vi "test_read-nmea-data2.vi"() -> ()   [LabVIEW 2019] (continued)
\n15:12:28.01\tF9P\t\t\n15:12:28.03\tF9P\t\t\n15:12:28.05\tF9P\t\t\n15:12:28.07\tF9P\t\t\n15:12:28.09\tF9P\t\t\n15:12:28.11\tF9P\t\t\n15:12:28.13\tF9P\t\t\n15:12:28.15\tF9P\t\t\n15:12:28.17\tF9P\t\t\n15:12:28.19\tF9P\t\t\n15:12:28.21\tF9P\t\t\n15:12:28.23\tF9P\t$GNRMC,061230.00,A,3723.54055,N,12656.94219,E,1.668,58.60,250720,,,A,V*39\n\t\n15:12:28.25\tF9P\t$GNVTG,58.60,T,,M,1.668,N,3.089,K,A*13\n\t\n15:12:28.27\tF9P\t$GNGGA,061230.00,3723.54055,N,12656.94219,E,1,12,0.92,43.1,M,18.5,M,,*73\n\t\n15:12:28.29\tF9P\t$GNGSA,A,3,12,06,19,05,17,09,04,02,,,,,1.52,0.92,1.22,1*0C\n\t\n15:12:28.31\tF9P\t$GNGSA,A,3,85,70,71,84,,,,,,,,,1.52,0.92,1.22,2*0E\n\t\n15:12:28.33\tF9P\t$GNGSA,A,3,36,19,11,04,09,12,,,,,,,1.52,0.92,1.22,3*0C\n\t\n15:12:28.35\tF9P\t$GNGSA,A,3,14,11,33,,,,,,,,,,1.52,0.92,1.22,4*0D\n\t\n15:12:28.37\tF9P\t$GPGSV,3,1,09,02,55,319,20,04,18,043,27,05,37,247,33,06,64,049,30,1*61\n\t\n15:12:28.39\tF9P\t$GPGSV,3,2,09,09,45,074,31,12,23,276,31,17,33,154,37,19,52,157,32,1*69\n\t\n15:12:28.41\tF9P\t$GPGSV,3,3,09,25,12,306,,1*5C\n\t\n15:12:28.43\tF9P\t$GPGSV,3,1,09,02,55,319,,04,18,043,21,05,37,247,26,06,64,049,26,6*61\n\t\n15:12:28.45\tF9P\t$GPGSV,3,2,09,09,45,074,25,12,23,276,17,17,33,154,31,19,52,157,,6*68\n\t\n15:12:28.47\tF9P\t$GPGSV,3,3,09,25,12,306,,6*5B\n\t\n15:12:28.49\tF9P\t$GLGSV,2,1,08,69,12,031,,70,71,039,28,71,52,205,42,72,04,209,24,1*70\n\t\n15:12:28.51\tF9P\t$GLGSV,2,2,08,77,01,326,,84,20,122,12,85,70,067,33,86,37,330,,1*7B\n\t\n15:12:28.53\tF9P\t$GLGSV,2,1,08,69,12,031,,70,71,039,,71,52,205,31,72,04,209,,3*7A\n\t\n15:12:28.55\tF9P\t$GLGSV,2,2,08,77,01,326,,84,20,122,11,85,70,067,25,86,37,330,,3*7D\n\t\n15:12:28.57\tF9P\t$GAGSV,2,1,08,02,08,297,11,04,66,116,29,09,32,193,33,11,71,358,32,7*7D\n\t\n15:12:28.59\tF9P\t$GAGSV,2,2,08,12,40,102,28,19,26,045,19,25,09,249,,36,26,308,15,7*7F\n\t\n15:12:28.61\tF9P\t$GAGSV,2,1,08,02,08,297,,04,66,116,,09,32,193,,11,71,358,,2*72\n\t\n15:12:28.63\tF9P\t$GAGSV,2,2,08,12,40,102,,19,26,045,,25,09,249,,36,26,308,,2*7C\n\t\n15:12:28.66\tF9P\t$GBGSV,1,1,04,11,50,132,34,14,87,127,32,28,,,18,33,60,219,37,1*44\n\t\n15:12:28.68\tF9P\t$GBGSV,1,1,03,11,50,132,31,14,87,127,,33,60,219,,3*42\n\t\n15:12:28.70\tF9P\t$GNGLL,3723.54055,N,12656.94219,E,061230.00,A,A*74\n\t\n15:12:28.72\tF9P\t\t\n15:12:28.74\tF9P\t\t\n15:12:28.76\tF9P\t\t\n15:12:28.78\tF9P\t\t\n15:12:28.80\tF9P\t\t\n15:12:28.82\tF9P\t\t\n15:12:28.84\tF9P\t\t\n15:12:28.86\tF9P\t\t\n15:12:28.88\tF9P\t\t\n15:12:28.90\tF9P\t\t\n15:12:28.92\tF9P\t\t\n15:12:28.94\tF9P\t\t\n15:12:28.96\tF9P\t\t\n15:12:28.98\tF9P\t\t\n15:12:29.00\tF9P\t\t\n15:12:29.02\tF9P\t\t\n15:12:29.04\tF9P\t\t\n15:12:29.06\tF9P\t\t\n15:12:29.08\tF9P\t\t\n15:12:29.10\tF9P\t\t\n15:12:29.12\tF9P\t\t\n15:12:29.14\tF9P\t\t\n15:12:29.16\tF9P\t\t\n15:12:29.18\tF9P\t\t\n15:12:29.20\tF9P\t\t\n15:12:29.22\tF9P\t\t\n15:12:29.24\tF9P\t$GNRMC,061231.00,A,3723.54087,N,12656.94280,E,1.630,70.48,250720,,,A,V*3A\n\t\n15:12:29.26\tF9P\t$GNVTG,70.48,T,,M,1.630,N,3.018,K,A*16\n\t\n15:12:29.28\tF9P\t$GNGGA,061231.00,3723.54087,N,12656.94280,E,1,12,0.75,42.3,M,18.5,M,,*77\n\t\n15:12:29.30\tF9P\t$GNGSA,A,3,12,06,19,05,17,09,04,02,,,,,1.29,0.75,1.04,1*0D\n\t\n15:12:29.32\tF9P\t$GNGSA,A,3,85,70,71,84,,,,,,,,,1.29,0.75,1.04,2*0F\n\t\n15:12:29.34\tF9P\t$GNGSA,A,3,36,19,11,04,09,12,,,,,,,1.29,0.75,1.04,3*0D\n\t\n15:12:29.36\tF9P\t$GNGSA,A,3,14,11,33,,,,,,,,,,1.29,0.75,1.04,4*0C\n\t\n15:12:29.38\tF9P\t$GPGSV,3,1,09,02,55,319,21,04,18,043,28,05,37,247,34,06,64,049,35,1*6D\n\t\n15:12:29.40\tF9P\t$GPGSV,3,2,09,09,45,074,32,12,23,276,27,17,33,154,37,19,52,157,31,1*6E\n\t\n15:12:29.42\tF9P\t$GPGSV,3,3,09,25,12,306,,1*5C\n\t\n15:12:29.44\tF9P\t$GPGSV,3,1,09,02,55,319,,04,18,043,22,05,37,247,27,06,64,049,26,6*63\n\t\n15:12:29.46\tF9P\t$GPGSV,3,2,09,09,45,074,25,12,23,276,17,17,33,154,31,19,52,157,,6*68\n\t\n15:12:29.48\tF9P\t$GPGSV,3,3,09,25,12,306,,6*5B\n\t\n15:12:29.50\tF9P\t$GLGSV,2,1,08,69,12,031,,70,71,039,33,71,52,205,32,72,04,209,25,1*7C\n\t\n15:12:29.52\tF9P\t$GLGSV,2,2,08,77,01,326,,84,20,122,12,85,70,067,33,86,37,330,,1*7B\n\t\n15:12:29.54\tF9P\t$GLGSV,2,1,08,69,12,031,,70,71,039,,71,52,205,26,72,04,209,,3*7C\n\t\n15:12:29.56\tF9P\t$GLGSV,2,2,08,77,01,326,,84,20,122,17,85,70,067,23,86,37,330,,3*7D\n\t\n15:12:29.58\tF9P\t$GAGSV,2,1,08,02,08,297,10,04,66,116,34,09,32,193,39,11,71,358,27,7*7E\n\t\n15:12:29.60\tF9P\t$GAGSV,2,2,08,12,40,102,27,19,26,045,19,25,09,249,,36,26,308,15,7*70\n\t\n15:12:29.62\tF9P\t$GAGSV,2,1,08,02,08,297,,04,66,116,,09,32,193,37,11,71,358,,2*76\n\t\n15:12:29.64\tF9P\t$GAGSV,2,2,08,12,40,102,,19,26,045,,25,09,249,,36,26,308,,2*7C\n\t\n15:12:29.66\tF9P\t$GBGSV,1,1,04,11,50,132,33,14,87,127,28,28,,,16,33,60,219,27,1*47\n\t\n15:12:29.68\tF9P\t$GBGSV,1,1,03,11,50,132,,14,87,127,29,33,60,219,,3*4B\n\t\n15:12:29.70\tF9P\t$GNGLL,3723.54087,N,12656.94280,E,061231.00,A,A*7A\n\t\n15:12:29.72\tF9P\t\t\n15:12:29.74\tF9P\t\t\n15:12:29.76\tF9P\t\t\n15:12:29.78\tF9P\t\t\n15:12:29.80\tF9P\t\t\n15:12:29.82\tF9P\t\t\n15:12:29.84\tF9P\t\t\n15:12:29.86\tF9P\t\t\n15:12:29.88\tF9P\t\t\n15:12:29.90\tF9P\t\t\n15:12:29.92\tF9P\t\t\n15:12:29.94\tF9P\t\t\n15:12:29.96\tF9P\t\t\n15:12:29.98\tF9P\t\t\n15:12:30.00\tF9P\t\t\n15:12:30.02\tF9P\t\t\n15:12:30.04\tF9P\t\t\n15:12:30.06\tF9P\t\t\n15:12:30.08\tF9P\t\t\n15:12:30.10\tF9P\t\t\n15:12:30.12\tF9P\t\t\n15:12:30.14\tF9P\t\t\n15:12:30.16\tF9P\t\t\n15:12:30.18\tF9P\t\t\n15:12:30.20\tF9P\t\t\n15:12:30.22\tF9P\t\t\n15:12:30.24\tF9P\t$GNRMC,061232.00,A,3723.54094,N,12656.94350,E,1.661,66.68,250720,,,A,V*36\n\t\n15:12:30.26\tF9P\t$GNVTG,66.68,T,,M,1.661,N,3.077,K,A*1E\n\t\n15:12:30.28\tF9P\t$GNGGA,061232.00,3723.54094,N,12656.94350,E,1,12,0.75,43.1,M,18.5,M,,*79\n\t\n15:12:30.30\tF9P\t$GNGSA,A,3,12,06,19,05,17,09,04,02,,,,,1.29,0.75,1.04,1*0D\n\t\n15:12:30.32\tF9P\t$GNGSA,A,3,85,70,71,84,,,,,,,,,1.29,0.75,1.04,2*0F\n\t\n15:12:30.34\tF9P\t$GNGSA,A,3,36,19,11,04,09,12,,,,,,,1.29,0.75,1.04,3*0D\n\t\n15:12:30.36\tF9P\t$GNGSA,A,3,14,11,33,,,,,,,,,,1.29,0.75,1.04,4*0C\n\t\n15:12:30.38\tF9P\t$GPGSV,3,1,09,02,55,319,21,04,18,043,28,05,37,247,40,06,64,049,32,1*69\n\t\n15:12:30.40\tF9P\t$GPGSV,3,2,09,09,45,074,32,12,23,276,27,17,33,154,38,19,52,157,32,1*62\n\t\n15:12:30.42\tF9P\t$GPGSV,3,3,09,25,12,306,,1*5C\n\t\n15:12:30.44\tF9P\t$GPGSV,3,1,09,02,55,319,,04,18,043,21,05,37,247,33,06,64,049,26,6*65\n\t\n15:12:30.46\tF9P\t$GPGSV,3,2,09,09,45,074,25,12,23,276,18,17,33,154,31,19,52,157,,6*67\n\t\n15:12:30.48\tF9P\t$GPGSV,3,3,09,25,12,306,,6*5B\n\t\n15:12:30.50\tF9P\t$GLGSV,2,1,08,69,12,031,,70,71,039,28,71,52,205,43,72,04,209,25,1*70\n\t\n15:12:30.52\tF9P\t$GLGSV,2,2,08,77,01,326,,84,20,122,11,85,70,067,36,86,37,330,,1*7D\n\t\n15:12:30.54\tF9P\t$GLGSV,2,1,08,69,12,031,,70,71,039,,71,52,205,25,72,04,209,,3*7F\n\t\n15:12:30.56\tF9P\t$GLGSV,2,2,08,77,01,326,,84,20,122,20,85,70,067,24,86,37,330,,3*7E\n\t\n15:12:30.58\tF9P\t$GAGSV,2,1,08,02,08,297,09,04,66,116,24,09,32,193,34,11,72,359,27,7*78\n\t\n15:12:30.60\tF9P\t$GAGSV,2,2,08,12,40,102,28,19,26,045,17,25,09,249,,36,26,308,15,7*71\n\t\n15:12:30.62\tF9P\t$GAGSV,2,1,08,02,08,297,,04,66,116,,09,32,193,,11,72,359,,2*70\n\t\n15:12:30.64\tF9P\t$GAGSV,2,2,08,12,40,102,,19,26,045,,25,09,249,,36,26,308,,2*7C\n\t\n15:12:30.66\tF9P\t$GBGSV,1,1,04,11,50,132,32,14,87,127,27,28,,,17,33,60,219,28,1*47\n\t\n15:12:30.68\tF9P\t$GBGSV,1,1,03,11,50,132,27,14,87,127,33,33,60,219,,3*45\n\t\n15:12:30.70\tF9P\t$GNGLL,3723.54094,N,12656.94350,E,061232.00,A,A*77\n\t\n15:12:30.72\tF9P\t\t\n15:12:30.74\tF9P\t\t\n15:12:30.76\tF9P\t\t\n15:12:30.78\tF9P\t\t\n15:12:30.80\tF9P\t\t\n15:12:30.82\tF9P\t\t\n15:12:30.84\tF9P\t\t\n15:12:30.86\tF9P\t\t\n15:12:30.88\tF9P\t\t\n15:12:30.90\tF9P\t\t\n15:12:30.92\tF9P\t\t\n15:12:30.94\tF9P\t\t\n15:12:30.96\tF9P\t\t\n15:12:30.98\tF9P\t\t\n15:12:31.00\tF9P\t\t\n15:12:31.02\tF9P\t\t\n15:12:31.04\tF9P\t\t\n15:12:31.06\tF9P\t\t\n15:12:31.08\tF9P\t\t\n15:12:31.10\tF9P\t\t\n15:12:31.12\tF9P\t\t\n15:12:31.14\tF9P\t\t\n15:12:31.16\tF9P\t\t\n15:12:31.18\tF9P\t\t\n15:12:31.20\tF9P\t\t\n15:12:31.22\tF9P\t\t\n15:12:31.24\tF9P\t$GNRMC,061233.00,A,3723.54127,N,12656.94381,E,1.460,37.45,250720,,,A,V*3A\n\t\n15:12:31.26\tF9P\t$GNVTG,37.45,T,,M,1.460,N,2.704,K,A*14\n\t\n15:12:31.28\tF9P\t$GNGGA,061233.00,3723.54127,N,12656.94381,E,1,12,0.75,43.9,M,18.5,M,,*75\n\t\n15:12:31.30\tF9P\t$GNGSA,A,3,12,06,19,05,17,09,04,02,,,,,1.29,0.75,1.04,1*0D\n\t\n15:12:31.32\tF9P\t$GNGSA,A,3,85,70,71,84,,,,,,,,,1.29,0.75,1.04,2*0F\n\t\n15:12:31.34\tF9P\t$GNGSA,A,3,36,19,11,04,09,12,,,,,,,1.29,0.75,1.04,3*0D\n\t\n15:12:31.36\tF9P\t$GNGSA,A,3,14,11,33,,,,,,,,,,1.29,0.75,1.04,4*0C\n\t\n15:12:31.38\tF9P\t$GPGSV,3,1,09,02,55,319,20,04,18,043,27,05,37,247,30,06,64,049,31,1*63\n\t\n15:12:31.40\tF9P\t$GPGSV,3,2,09,09,45,074,32,12,23,276,27,17,33,154,28,19,52,157,28,1*68\n\t\n15:12:31.42\tF9P\t$GPGSV,3,3,09,25,12,306,,1*5C\n\t\n15:12:31.44\tF9P\t$GPGSV,3,1,09,02,55,319,,04,18,043,23,05,37,247,28,06,64,049,25,6*6E\n\t\n15:12:31.46\tF9P\t$GPGSV,3,2,09,09,45,074,31,12,23,276,17,17,33,154,26,19,52,157,,6*6B\n\t\n15:12:31.48\tF9P\t$GPGSV,3,3,09,25,12,306,,6*5B\n\t\n15:12:31.50\tF9P\t$GLGSV,2,1,08,69,12,031,,70,71,039,28,71,52,205,43,72,04,209,25,1*70\n\t\n15:12:31.52\tF9P\t$GLGSV,2,2,08,77,01,326,,84,20,122,12,85,70,067,34,86,37,330,,1*7C\n\t\n15:12:31.54\tF9P\t$GLGSV,2,1,08,69,12,031,,70,71,039,,71,52,205,26,72,04,209,,3*7C\n\t\n15:12:31.56\tF9P\t$GLGSV,2,2,08,77,01,326,,84,20,122,18,85,70,067,24,86,37,330,,3*75\n\t\n15:12:31.58\tF9P\t$GAGSV,2,1,08,02,08,297,10,04,66,116,26,09,32,193,29,11,72,359,33,7*7B\n\t\n15:12:31.60\tF9P\t$GAGSV,2,2,08,12,40,103,29,19,26,045,17,25,09,249,,36,26,308,15,7*71\n\t\n15:12:31.62\tF9P\t$GAGSV,2,1,08,02,08,297,,04,66,116,,09,32,193,,11,72,359,,2*70\n\t\n15:12:31.64\tF9P\t$GAGSV,2,2,08,12,40,103,,19,26,045,,25,09,249,,36,26,308,,2*7D\n\t\n15:12:31.66\tF9P\t$GBGSV,1,1,04,11,50,132,31,14,87,127,31,28,,,17,33,60,219,33,1*49\n\t\n15:12:31.68\tF9P\t$GBGSV,1,1,03,11,50,132,29,14,87,127,29,33,60,219,,3*40\n\t\n15:12:31.70\tF9P\t$GNGLL,3723.54127,N,12656.94381,E,061233.00,A,A*73\n\t\n15:12:31.72\tF9P\t\t\n15:12:31.74\tF9P\t\t\n15:12:31.76\tF9P\t\t\n15:12:31.78\tF9P\t\t\n15:12:31.80\tF9P\t\t\n15:12:31.82\tF9P\t\t\n15:12:31.84\tF9P\t\t\n15:12:31.86\tF9P\t\t\n15:12:31.88\tF9P\t\t\n15:12:31.90\tF9P\t\t\n15:12:31.92\tF9P\t\t\n15:12:31.94\tF9P\t\t\n15:12:31.96\tF9P\t\t\n15:12:31.98\tF9P\t\t\n15:12:32.00\tF9P\t\t\n15:12:32.02\tF9P\t\t\n15:12:32.04\tF9P\t\t\n15:12:32.06\tF9P\t\t\n15:12:32.08\tF9P\t\t\n15:12:32.10\tF9P\t\t\n15:12:32.12\tF9P\t\t\n15:12:32.14\tF9P\t\t\n15:12:32.16\tF9P\t\t\n15:12:32.18\tF9P\t\t\n15:12:32.20\tF9P\t\t\n15:12:32.22\tF9P\t\t\n15:12:32.24\tF9P\t$GNRMC,061234.00,A,3723.54165,N,12656.94434,E,2.294,54.61,250720,,,A,V*3F\n\t\n15:12:32.26\tF9P\t$GNVTG,54.61,T,,M,2.294,N,4.248,K,A*12\n\t\n15:12:32.28\tF9P\t$GNGGA,061234.00,3723.54165,N,12656.94434,E,1,12,0.86,45.3,M,18.5,M,,*7D\n\t\n15:12:32.30\tF9P\t$GNGSA,A,3,12,06,19,05,17,09,04,02,,,,,1.43,0.86,1.14,1*0C\n\t\n15:12:32.32\tF9P\t$GNGSA,A,3,85,70,71,84,,,,,,,,,1.43,0.86,1.14,2*0E\n\t\n15:12:32.34\tF9P\t$GNGSA,A,3,36,19,11,04,09,12,,,,,,,1.43,0.86,1.14,3*0C\n\t\n15:12:32.36\tF9P\t$GNGSA,A,3,14,11,33,,,,,,,,,,1.43,0.86,1.14,4*0D\n\t\n15:12:32.38\tF9P\t$GPGSV,3,1,09,02,55,319,20,04,18,043,26,05,37,247,35,06,64,049,33,1*65\n\t\n15:12:32.40\tF9P\t$GPGSV,3,2,09,09,45,074,36,12,23,276,27,17,33,154,34,19,52,157,33,1*6B\n\t\n15:12:32.42\tF9P\t$GPGSV,3,3,09,25,12,306,,1*5C\n\t\n15:12:32.44\tF9P\t$GPGSV,3,1,09,02,55,319,,04,18,043,20,05,37,247,26,06,64,049,25,6*63\n\t\n15:12:32.46\tF9P\t$GPGSV,3,2,09,09,45,074,31,12,23,276,18,17,33,154,26,19,52,157,,6*64\n\t\n15:12:32.48\tF9P\t$GPGSV,3,3,09,25,12,306,,6*5B\n\t\n15:12:32.50\tF9P\t$GLGSV,2,1,08,69,12,031,,70,71,039,33,71,52,205,40,72,04,209,25,1*79\n\t\n15:12:32.52\tF9P\t$GLGSV,2,2,08,77,01,326,,84,20,122,09,85,70,067,27,86,37,330,,1*74\n\t\n15:12:32.54\tF9P\t$GLGSV,2,1,08,69,12,031,,70,71,039,,71,52,205,27,72,04,209,,3*7D\n\t\n15:12:32.56\tF9P\t$GLGSV,2,2,08,77,01,326,,84,20,122,16,85,70,067,23,86,37,330,,3*7C\n\t\n15:12:32.58\tF9P\t$GAGSV,2,1,08,02,08,297,08,04,66,116,27,09,32,193,41,11,72,359,35,7*7B\n\t\n15:12:32.60\tF9P\t$GAGSV,2,2,08,12,40,103,28,19,26,045,15,25,09,249,,36,26,308,14,7*73\n\t\n15:12:32.62\tF9P\t$GAGSV,2,1,08,02,08,297,,04,66,116,,09,32,193,33,11,72,359,,2*70\n\t\n15:12:32.64\tF9P\t$GAGSV,2,2,08,12,40,103,,19,26,045,,25,09,249,,36,26,308,,2*7D\n\t\n15:12:32.66\tF9P\t$GBGSV,1,1,04,11,50,132,33,14,87,127,24,28,,,17,33,60,219,32,1*4E\n\t\n15:12:32.68\tF9P\t$GBGSV,1,1,03,11,50,132,36,14,87,127,33,33,60,219,,3*45\n\t\n15:12:32.70\tF9P\t$GNGLL,3723.54165,N,12656.94434,E,061234.00,A,A*7B\n\t\n15:12:32.72\tF9P\t\t\n15:12:32.74\tF9P\t\t\n15:12:32.76\tF9P\t\t\n15:12:32.78\tF9P\t\t\n15:12:32.80\tF9P\t\t\n15:12:32.82\tF9P\t\t\n15:12:32.84\tF9P\t\t\n15:12:32.86\tF9P\t\t\n15:12:32.88\tF9P\t\t\n15:12:32.90\tF9P\t\t\n15:12:32.92\tF9P\t\t\n15:12:32.94\tF9P\t\t\n15:12:32.96\tF9P\t\t\n15:12:32.98\tF9P\t\t\n15:12:33.00\tF9P\t\t\n15:12:33.02\tF9P\t\t\n15:12:33.04\tF9P\t\t\n15:12:33.06\tF9P\t\t\n15:12:33.08\tF9P\t\t\n15:12:33.10\tF9P\t\t\n15:12:33.12\tF9P\t\t\n15:12:33.14\tF9P\t\t\n15:12:33.16\tF9P\t\t\n15:12:33.18\tF9P\t\t\n15:12:33.20\tF9P\t\t\n15:12:33.22\tF9P\t\t\n15:12:33.24\tF9P\t$GNRMC,061235.00,A,3723.54212,N,12656.94529,E,2.410,59.12,250720,,,A,V*33\n\t\n15:12:33.26\tF9P\t$GNVTG,59.12,T,,M,2.410,N,4.463,K,A*1E\n\t\n15:12:33.28\tF9P\t$GNGGA,061235.00,3723.54212,N,12656.94529,E,1,12,0.86,45.6,M,18.5,M,,*77\n\t\n15:12:33.30\tF9P\t$GNGSA,A,3,12,06,19,05,17,09,04,02,,,,,1.43,0.86,1.14,1*0C\n\t\n15:12:33.32\tF9P\t$GNGSA,A,3,85,70,71,84,,,,,,,,,1.43,0.86,1.14,2*0E\n\t\n15:12:33.34\tF9P\t$GNGSA,A,3,36,19,11,04,09,12,,,,,,,1.43,0.86,1.14,3*0C\n\t\n15:12:33.36\tF9P\t$GNGSA,A,3,14,11,33,,,,,,,,,,1.43,0.86,1.14,4*0D\n\t\n15:12:33.38\tF9P\t$GPGSV,3,1,09,02,55,319,21,04,18,043,25,05,37,247,35,06,64,049,30,1*64\n\t\n15:12:33.40\tF9P\t$GPGSV,3,2,09,09,45,074,34,12,23,276,25,17,33,154,30,19,52,157,34,1*68\n\t\n15:12:33.42\tF9P\t$GPGSV,3,3,09,25,12,306,,1*5C\n\t\n15:12:33.44\tF9P\t$GPGSV,3,1,09,02,55,319,,04,18,043,19,05,37,247,27,06,64,049,31,6*6D\n\t\n15:12:33.46\tF9P\t$GPGSV,3,2,09,09,45,074,30,12,23,276,16,17,33,154,26,19,52,157,,6*6B\n\t\n15:12:33.48\tF9P\t$GPGSV,3,3,09,25,12,306,,6*5B\n\t\n15:12:33.50\tF9P\t$GLGSV,2,1,08,69,12,031,,70,71,039,33,71,52,205,41,72,04,209,25,1*78\n\t\n15:12:33.52\tF9P\t$GLGSV,2,2,08,77,01,326,,84,20,122,10,85,70,067,37,86,37,330,,1*7D\n\t\n15:12:33.54\tF9P\t$GLGSV,2,1,08,69,12,031,,70,71,039,,71,52,205,25,72,04,209,,3*7F\n\t\n15:12:33.56\tF9P\t$GLGSV,2,2,08,77,01,326,,84,20,122,17,85,70,067,23,86,37,330,,3*7D\n\t\n15:12:33.58\tF9P\t$GAGSV,2,1,08,02,08,297,13,04,66,116,28,09,32,193,30,11,72,359,32,7*7F\n\t\n15:12:33.60\tF9P\t$GAGSV,2,2,08,12,40,103,33,19,26,045,15,25,09,249,,36,26,308,14,7*79\n\t\n15:12:33.62\tF9P\t$GAGSV,2,1,08,02,08,297,,04,66,116,,09,32,193,35,11,72,359,,2*76\n\t\n15:12:33.64\tF9P\t$GAGSV,2,2,08,12,40,103,,19,26,045,,25,09,249,,36,26,308,,2*7D\n\t\n15:12:33.66\tF9P\t$GBGSV,1,1,04,11,50,132,25,14,87,127,25,28,,,19,33,60,219,36,1*42\n\t\n15:12:33.68\tF9P\t$GBGSV,1,1,03,11,50,132,,14,87,127,29,33,60,219,,3*4B\n\t\n15:12:33.70\tF9P\t$GNGLL,3723.54212,N,12656.94529,E,061235.00,A,A*74\n\t\n15:12:33.72\tF9P\t\t\n15:12:33.74\tF9P\t\t\n15:12:33.76\tF9P\t\t\n15:12:33.78\tF9P\t\t\n15:12:33.80\tF9P\t\t\n15:12:33.82\tF9P\t\t\n15:12:33.84\tF9P\t\t\n15:12:33.86\tF9P\t\t\n15:12:33.88\tF9P\t\t\n15:12:33.90\tF9P\t\t\n15:12:33.92\tF9P\t\t\n15:12:33.94\tF9P\t\t\n15:12:33.96\tF9P\t\t\n15:12:33.98\tF9P\t\t\n15:12:34.00\tF9P\t\t\n15:12:34.02\tF9P\t\t\n15:12:34.04\tF9P\t\t\n15:12:34.06\tF9P\t\t\n15:12:34.08\tF9P\t\t\n15:12:34.10\tF9P\t\t\n15:12:34.12\tF9P\t\t\n15:12:34.14\tF9P\t\t\n15:12:34.16\tF9P\t\t\n15:12:34.18\tF9P\t\t\n15:12:34.20\tF9P\t\t\n15:12:34.22\tF9P\t\t\n15:12:34.24\tF9P\t$GNRMC,061236.00,A,3723.54267,N,12656.94619,E,2.463,58.89,250720,,,A,V*35\n\t\n15:12:34.26\tF9P\t$GNVTG,58.89,T,,M,2.463,N,4.561,K,A*1A\n\t\n15:12:34.28\tF9P\t$GNGGA,061236.00,3723.54267,N,12656.94619,E,1,12,0.89,45.7,M,18.5,M,,*78\n\t\n15:12:34.30\tF9P\t$GNGSA,A,3,12,06,19,05,17,09,04,02,,,,,1.49,0.89,1.20,1*0E\n\t\n15:12:34.32\tF9P\t$GNGSA,A,3,85,70,71,84,,,,,,,,,1.49,0.89,1.20,2*0C\n\t\n15:12:34.34\tF9P\t$GNGSA,A,3,36,19,11,04,09,12,,,,,,,1.49,0.89,1.20,3*0E\n\t\n15:12:34.36\tF9P\t$GNGSA,A,3,14,11,33,,,,,,,,,,1.49,0.89,1.20,4*0F\n\t\n15:12:34.38\tF9P\t$GPGSV,3,1,09,02,55,319,22,04,18,043,25,05,37,247,32,06,64,049,29,1*68\n\t\n15:12:34.40\tF9P\t$GPGSV,3,2,09,09,45,074,35,12,23,276,25,17,33,154,29,19,52,157,29,1*6D\n\t\n15:12:34.42\tF9P\t$GPGSV,3,3,09,25,12,306,,1*5C\n\t\n15:12:34.44\tF9P\t$GPGSV,3,1,09,02,55,319,,04,18,043,19,05,37,247,26,06,64,049,31,6*6C\n\t\n15:12:34.46\tF9P\t$GPGSV,3,2,09,09,45,074,24,12,23,276,14,17,33,154,26,19,52,157,,6*6C\n\t\n15:12:34.48\tF9P\t$GPGSV,3,3,09,25,12,306,,6*5B\n\t\n15:12:34.50\tF9P\t$GLGSV,2,1,08,69,12,031,,70,71,039,32,71,52,205,44,72,04,209,26,1*7F\n\t\n15:12:34.52\tF9P\t$GLGSV,2,2,08,77,01,326,,84,20,122,09,85,70,067,39,86,37,330,,1*7B\n\t\n15:12:34.54\tF9P\t$GLGSV,2,1,08,69,12,031,,70,71,039,,71,52,205,25,72,04,209,,3*7F\n\t\n15:12:34.56\tF9P\t$GLGSV,2,2,08,77,01,326,,84,20,122,15,85,70,067,22,86,37,330,,3*7E\n\t\n15:12:34.58\tF9P\t$GAGSV,2,1,08,02,08,297,06,04,66,116,32,09,32,193,35,11,72,359,32,7*75\n\t\n15:12:34.60\tF9P\t$GAGSV,2,2,08,12,40,103,26,19,26,045,14,25,09,249,,36,26,308,17,7*7F\n\t\n15:12:34.62\tF9P\t$GAGSV,2,1,08,02,08,297,,04,66,116,,09,32,193,,11,72,359,,2*70\n\t\n15:12:34.64\tF9P\t$GAGSV,2,2,08,12,40,103,,19,26,045,,25,09,249,,36,26,308,,2*7D\n\t\n15:12:34.66\tF9P\t$GBGSV,1,1,04,11,50,132,31,14,87,127,30,28,,,21,33,60,219,36,1*48\n\t\n15:12:34.68\tF9P\t$GBGSV,1,1,03,11,50,132,,14,87,127,30,33,60,219,,3*43\n\t\n15:12:34.70\tF9P\t$GNGLL,3723.54267,N,12656.94619,E,061236.00,A,A*75\n\t\n15:12:34.72\tF9P\t\t\n15:12:34.75\tF9P\t\t\n15:12:34.77\tF9P\t\t\n15:12:34.79\tF9P\t\t\n15:12:34.81\tF9P\t\t\n15:12:34.83\tF9P\t\t\n15:12:34.85\tF9P\t\t\n15:12:34.87\tF9P\t\t\n15:12:34.89\tF9P\t\t\n15:12:34.91\tF9P\t\t\n15:12:34.93\tF9P\t\t\n15:12:34.95\tF9P\t\t\n15:12:34.97\tF9P\t\t\n15:12:34.99\tF9P\t\t\n15:12:35.01\tF9P\t\t\n15:12:35.03\tF9P\t\t\n15:12:35.05\tF9P\t\t\n15:12:35.07\tF9P\t\t\n15:12:35.09\tF9P\t\t\n15:12:35.11\tF9P\t\t\n15:12:35.13\tF9P\t\t\n15:12:35.15\tF9P\t\t\n15:12:35.17\tF9P\t\t\n15:12:35.19\tF9P\t\t\n15:12:35.21\tF9P\t\t\n15:12:35.23\tF9P\t$GNRMC,061237.00,A,3723.54317,N,12656.94702,E,2.443,57.94,250720,,,A,V*38\n\t\n15:12:35.25\tF9P\t$GNVTG,57.94,T,,M,2.443,N,4.524,K,A*1A\n\t\n15:12:35.27\tF9P\t$GNGGA,061237.00,3723.54317,N,12656.94702,E,1,12,0.86,46.6,M,18.5,M,,*79\n\t\n15:12:35.29\tF9P\t$GNGSA,A,3,12,06,19,05,17,09,04,02,,,,,1.43,0.86,1.14,1*0C\n\t\n15:12:35.31\tF9P\t$GNGSA,A,3,85,70,71,84,,,,,,,,,1.43,0.86,1.14,2*0E\n\t\n15:12:35.33\tF9P\t$GNGSA,A,3,36,19,11,04,09,12,,,,,,,1.43,0.86,1.14,3*0C\n\t\n15:12:35.35\tF9P\t$GNGSA,A,3,14,11,33,,,,,,,,,,1.43,0.86,1.14,4*0D\n\t\n15:12:35.37\tF9P\t$GPGSV,3,1,09,02,55,319,21,04,18,043,24,05,37,247,31,06,64,049,27,1*67\n\t\n15:12:35.39\tF9P\t$GPGSV,3,2,09,09,45,074,26,12,23,276,31,17,33,154,32,19,52,157,30,1*68\n\t\n15:12:35.41\tF9P\t$GPGSV,3,3,09,25,12,306,,1*5C\n\t\n15:12:35.43\tF9P\t$GPGSV,3,1,09,02,55,319,,04,18,043,18,05,37,247,23,06,64,049,28,6*60\n\t\n15:12:35.45\tF9P\t$GPGSV,3,2,09,09,45,074,30,12,23,276,15,17,33,154,25,19,52,157,,6*6B\n\t\n15:12:35.47\tF9P\t$GPGSV,3,3,09,25,12,306,,6*5B\n\t\n15:12:35.49\tF9P\t$GLGSV,2,1,08,69,12,031,,70,71,039,32,71,52,205,35,72,04,209,26,1*79\n\t\n15:12:35.51\tF9P\t$GLGSV,2,2,08,77,01,326,,84,20,122,10,85,70,067,40,86,37,330,,1*7D\n\t\n15:12:35.53\tF9P\t$GLGSV,2,1,08,69,12,031,,70,71,039,,71,52,205,25,72,04,209,,3*7F\n\t\n15:12:35.55\tF9P\t$GLGSV,2,2,08,77,01,326,,84,20,122,14,85,70,067,22,86,37,330,,3*7F\n\t\n15:12:35.57\tF9P\t$GAGSV,2,1,08,02,08,297,09,04,66,116,27,09,32,193,35,11,72,359,27,7*7A\n\t\n15:12:35.59\tF9P\t$GAGSV,2,2,08,12,40,103,19,19,26,045,17,25,09,249,,36,26,308,19,7*7E\n\t\n15:12:35.61\tF9P\t$GAGSV,2,1,08,02,08,297,,04,66,116,,09,32,193,,11,72,359,,2*70\n\t\n15:12:35.63\tF9P\t$GAGSV,2,2,08,12,40,103,,19,26,045,,25,09,249,,36,26,308,,2*7D\n\t\n15:12:35.65\tF9P\t$GBGSV,1
